vi "CalibrationVolumes.vi"() -> ()   [LabVIEW 2013]
panel:
  out "AllCalibrationVolumes":T1(array[cluster]) {"CalibrationVolumes" format="%.6g"}
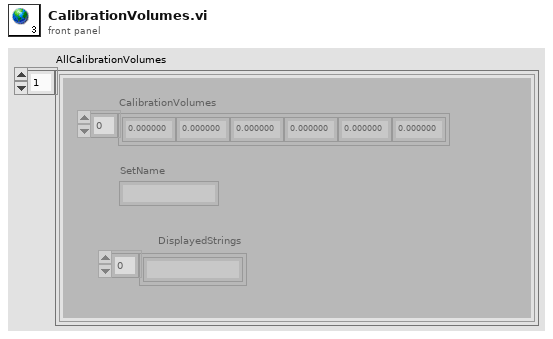
[diagram p1: front panel]
types:
  T1 = cluster{"CalibrationVolumes":dbl[], "SetName":string, "DisplayedStrings":string[]}[]
diagram:
